vi "AR-Log-gas-cycle.vi"(8 "error in":errorcluster, 10 "Log Data":T1 {"O2 Timer" format="%.1f sec"; "Gas sol timer" format="%.1f sec"; "Vac sol timer" format="%.1f sec"; "O2 1000ppm (AI3)" format="%.0f PPM"; "0-25% O2 (AI2)" format="%.2f %"; "1000 Torr (AI1)" format="%.2f Torr"; "10 Torr (AI0)" format="%.3f Torr"}, 11 "Path to Save Report":path=path "C:/Users/cleanroom/Desktop/Gas-cycle-logs/Report-1-11-22") -> (0 "error out":errorcluster, 3 "Log Written":bool)   [LabVIEW 2021]
doc: "Saves a .csv file with the test values plus a header with all user input information."
uses:
  Controls/AR-log-data-gas-cycle.ctl
  <vilib>/Utility/error.llb/whitespace.ctl
panel:
  out "Results Log":string="1,A,1,SB,1.023,1.050,2,2.345,2.500,10,Fail\r1,A,1,SB,1.023,1.050,2,2.345,2.500,10,Pass\r"
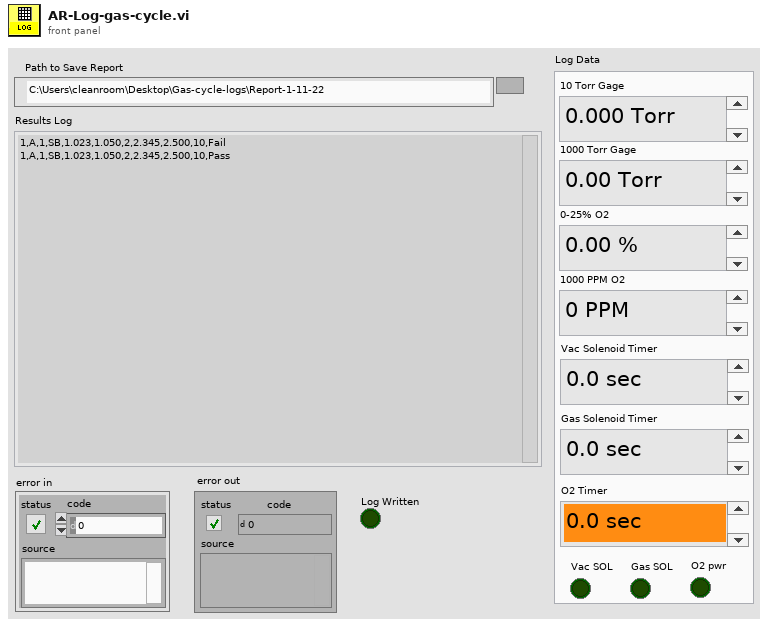
[diagram p1: front panel]
types:
  T1 = typedef "AR-log-data-gas-cycle.ctl" = cluster{"10 Torr (AI0)":dbl, "1000 Torr (AI1)":dbl, "0-25% O2 (AI2)":dbl, "O2 1000ppm (AI3)":dbl, "Vac sol timer":dbl, "Gas sol timer":dbl, "O2 Timer":dbl, "Vac SOL":bool, "Gas SOL":bool, "O2 pwr":bool}
  T2 = typedef "whitespace.ctl" = u16
  T3 = enum16{"open", "replace", "create", "open or create", "replace or create", "replace or create with confirmation"}
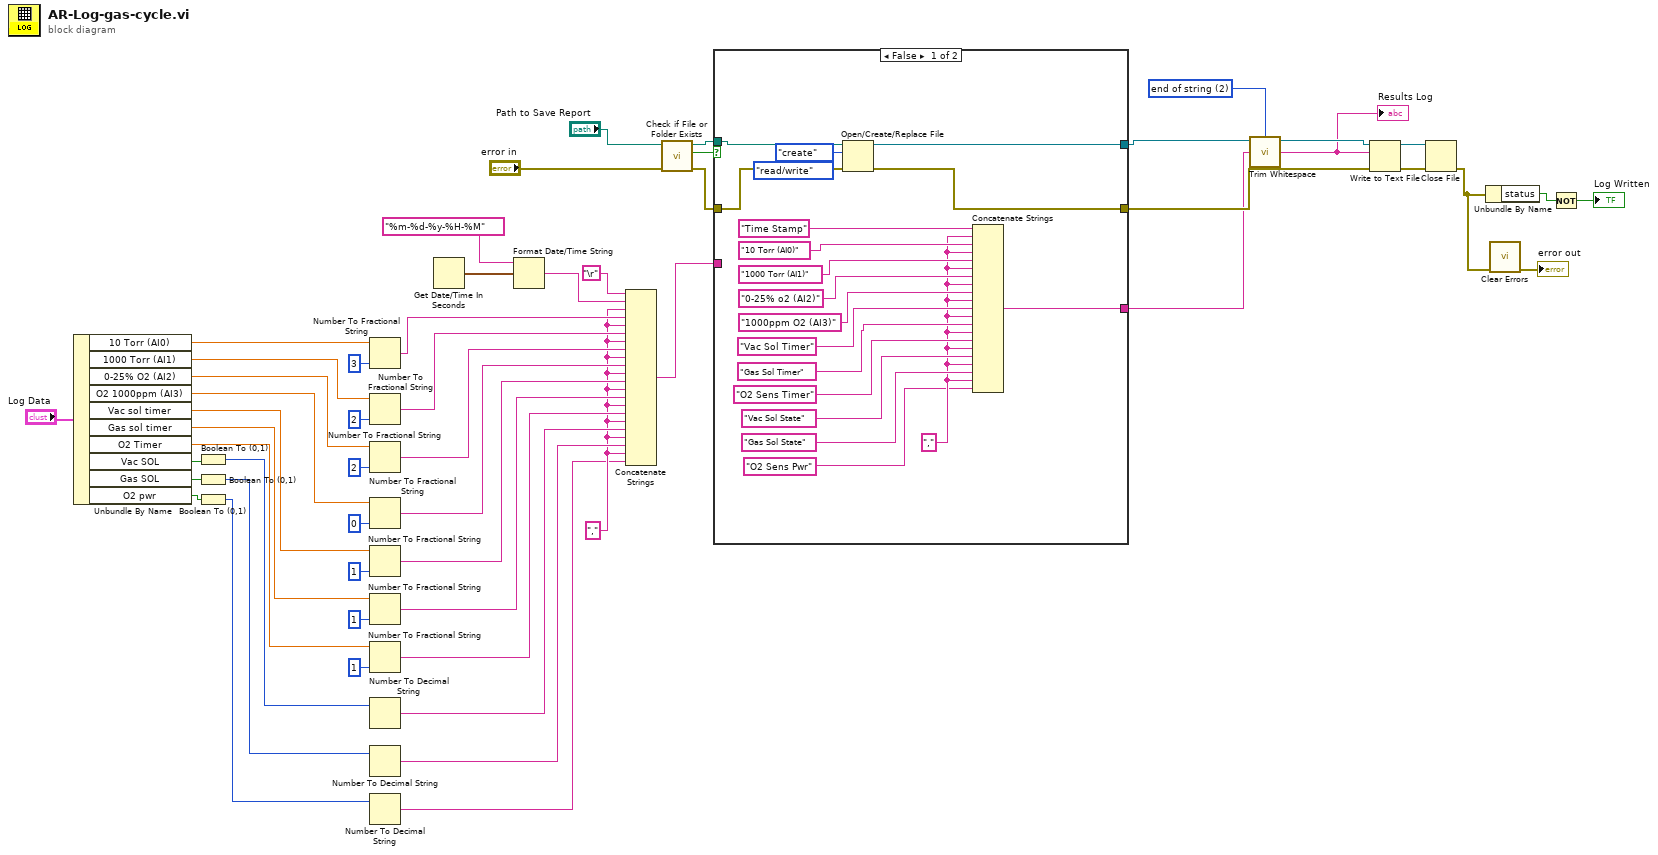
[diagram p0: block diagram]
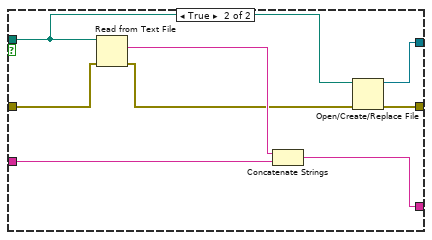
[diagram p2: hidden frame]
diagram:
  w2 = ","
  w44 = T2 2 items=["both", "start of string", "end of string"] ("location (both)")
  n1 = Unbundle By Name("Log Data") -> ("10 Torr (AI0)"=w37:dbl, "1000 Torr (AI1)"=w35:dbl, "0-25% O2 (AI2)"=w30:dbl, "O2 1000ppm (AI3)"=w31:dbl, "Vac sol timer"=w8:dbl, "Gas sol timer"=w9:dbl, "O2 Timer"=w10:dbl, "Vac SOL"=w17:bool, "Gas SOL"=w16:bool, "O2 pwr"=w15:bool)
  n2 = Boolean To (0,1)(Boolean=w17) -> (0, 1=w11:i16)
  n3 = Boolean To (0,1)(Boolean=w16) -> (0, 1=w12:i16)
  n4 = Boolean To (0,1)(Boolean=w15) -> (0, 1=w13:i16)
  n5 = Number To Fractional String(number=w37, precision (6)=i16 3) -> (F-format string=w29:string)  [unwired: 2 in]
  n6 = Number To Fractional String(number=w35, precision (6)=i16 2) -> (F-format string=w28:string)  [unwired: 2 in]
  n7 = Number To Fractional String(number=w30, precision (6)=i16 2) -> (F-format string=w27:string)  [unwired: 2 in]
  n8 = Number To Fractional String(number=w31, precision (6)=i16 0) -> (F-format string=w26:string)  [unwired: 2 in]
  n9 = Number To Fractional String(number=w8, precision (6)=i16 1) -> (F-format string=w7:string)  [unwired: 2 in]
  n10 = Number To Fractional String(number=w9, precision (6)=i16 1) -> (F-format string=w6:string)  [unwired: 2 in]
  n11 = Number To Fractional String(number=w10, precision (6)=i16 1) -> (F-format string=w5:string)  [unwired: 2 in]
  n12 = Number To Decimal String(number=w11) -> (decimal integer string=w4:string)  [unwired: 1 in]
  n13 = Number To Decimal String(number=w12) -> (decimal integer string=w3:string)  [unwired: 1 in]
  n14 = Number To Decimal String(number=w13) -> (decimal integer string=w1:string)  [unwired: 1 in]
  n15 = Get Date/Time In Seconds() -> (seconds since 1Jan1904=w52:timestamp)
  n16 = Format Date/Time String(time format string (%c)="%m-%d-%y-%H-%M", seconds (now)=w52) -> (date/time string=w39:string)  [unwired: 1 in]
  n17 = Concatenate Strings("\r", w39, w2, w29, w2, w28, w2, w27, w2, w26, w2, w7, w2, w6, w2, w5, w2, w4, w2, w3, w2, w1) -> (w50:string)
  n18 = call <vilib>:"Check if File or Folder Exists.vi"("error in (no error)"="error in", "path"="Path to Save Report") -> ("error out"=w47:errorcluster, "file or folder exists?"=w49:bool, "dup path"=w48:path)  [unwired: 7 in]
  n19 = case shown="False" w49 {
    tunnel: [w63 w74] -> w41
    tunnel: [w65 w73] -> w43
    tunnel: w48 -> [w64 w75]
    tunnel: w47 -> [w66 w80]
    tunnel: w50 -> [_ w78]
    tunnel: [w67 w77] -> w25
    frame False {
      w55 = ","
      n20 = Open/Create/Replace File(file path (use dialog)=w64, error in=w66, operation (0:open)=T3."create", access (0:read/write)=enum16{"read/write", "read-only", "write-only"}."read/write") -> (refnum out=w63:refnum<file>, error out=w65:errorcluster)  [unwired: 2 in, 1 out]
      n21 = Concatenate Strings("Time Stamp" ("string"), w55, "10 Torr (AI0)" ("string"), w55, "1000 Torr (AI1)" ("string"), w55, "0-25% o2 (AI2)" ("string"), w55, "1000ppm O2 (AI3)" ("string"), w55, "Vac Sol Timer" ("string"), w55, "Gas Sol Timer" ("string"), w55, "O2 Sens Timer" ("string"), w55, "Vac Sol State" ("string"), w55, "Gas Sol State" ("string"), w55, "O2 Sens Pwr" ("string")) -> (w67:string)
    }
    frame True {
      n22 = Read from Text File(file (use dialog)=w75, error in=w80) -> (text=w79:string, error out=w76:errorcluster)  [unwired: 2 in, 2 out]
      n23 = Concatenate Strings(w79, w78) -> (w77:string)
      n24 = Open/Create/Replace File(file path (use dialog)=w75, error in=w76) -> (refnum out=w74:refnum<file>, error out=w73:errorcluster)  [unwired: 4 in, 1 out]
    }
  }
  n25 = call <vilib>:"Trim Whitespace.vi"("string"=w25, "location (both)"=w44) -> ("trimmed string"=w24:string)
  "Results Log" <- w24
  n26 = Write to Text File(file (use dialog)=w41, text=w24, error in=w43) -> (refnum out=w45:refnum<file>, error out=w46:errorcluster)  [unwired: 1 in, 1 out]
  n27 = Close File(refnum=w45, error in=w46) -> (error out=w20:errorcluster)  [unwired: 1 out]
  n28 = Unbundle By Name(w20) -> ("status"=w23:bool)
  n29 = call <vilib>:"Clear Errors.vi"("error in (no error)"=w20) -> ("error out"=→"error out":errorcluster)  [unwired: 5 in, 1 out]
  n30 = Not(x=w23) -> (.not. x?=→"Log Written":bool)
